vi "GetVariantToDataError.vi"(10 "error close reference":errorcluster, 11 "server":T1={"vi name"="", "VI Refnum"=refnum, "queue"=refnum, "ROS"={"topic port"=0, "Node"="", "topic"="", "type"="", "node port"=0, "error "={"status"=FALSE, "code"=0, "source"=""}, "Direction"=enum."Node", "APIs"=[], "Update (ms)"=1, "write queue"=1}, "notifier"=refnum}) -> ()   [LabVIEW 2012]
uses:
  <userlib>/ROSforLV/ROS/Code/Console/Servers/ServerSubs/ServoInfo.ctl
  <userlib>/ROSforLV/ROS/Code/SubVIs/_ROSControl.ctl
  <userlib>/ROSforLV/ROS/Code/SubVIs/_ROSDirection.ctl
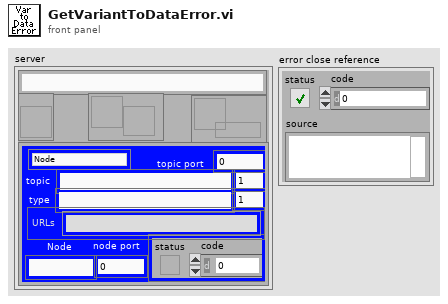
[diagram p1: front panel]
types:
  T1 = typedef "ServoInfo.ctl" = cluster{"vi name":string, "VI Refnum":refnum<vi>, "queue":refnum<queue>, "ROS":T2, "notifier":refnum<notifier>}
  T2 = typedef "_ROSControl.ctl" = cluster{"topic port":u16, "Node":string, "topic":string, "type":string, "node port":u16, "error ":errorcluster, "Direction":T3, "APIs":string[], "Update (ms)":u16, "write queue":u16}
  T3 = typedef "_ROSDirection.ctl" = enum16{"Node", "Publisher", "Subscriber", "Service Client"}
  T4 = enum16{"open", "replace", "create", "open or create", "replace or create", "replace or create with confirmation"}
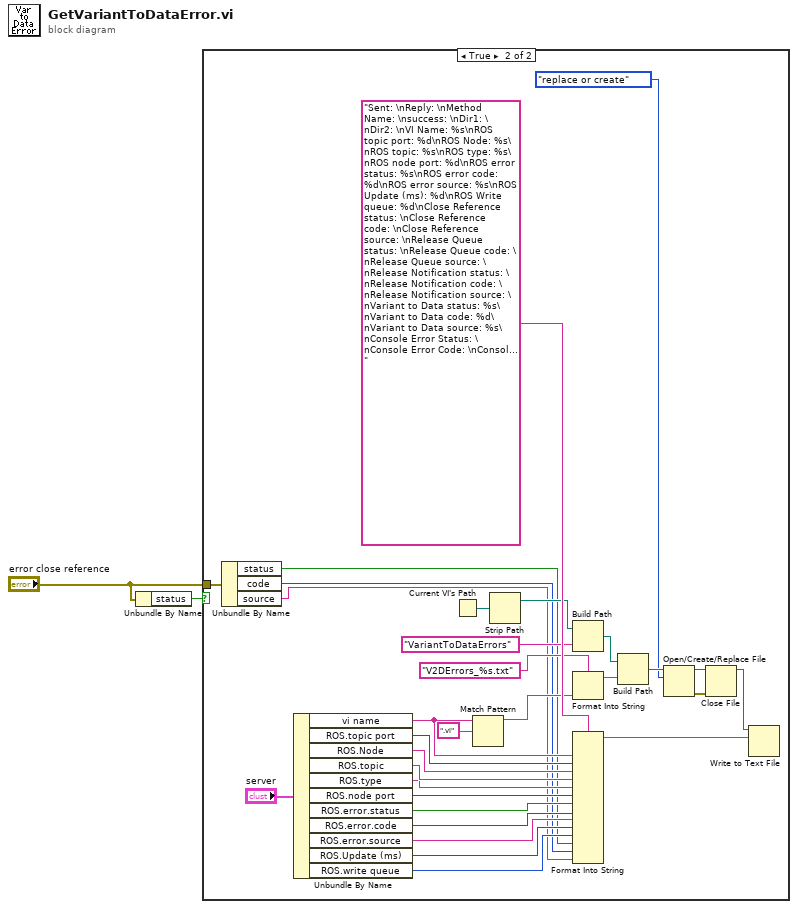
[diagram p0: block diagram]
diagram:
  n1 = Unbundle By Name("error close reference") -> ("status"=w2:bool)
  n2 = case shown="True" w2 {
    tunnel: "error close reference" -> [_ w17]
    frame False {
    }
    frame True {
      n3 = Unbundle By Name(w17) -> ("status"=w5:bool, "code"=w4:i32, "source"=w3:string)
      n4 = Unbundle By Name("server") -> ("vi name"=w16:string, "ROS.topic port"=w15:u16, "ROS.Node"=w14:string, "ROS.topic"=w13:string, "ROS.type"=w12:string, "ROS.node port"=w11:u16, "ROS.error.status"=w10:bool, "ROS.error.code"=w9:i32, "ROS.error.source"=w8:string, "ROS.Update (ms)"=w7:u16, "ROS.write queue"=w6:u16)
      n5 = Current VI's Path() -> (path=w31:path)
      n6 = Match Pattern(string=w16, regular expression=".vi") -> (before substring=w18:string)  [unwired: 1 in, 3 out]
      n7 = Strip Path(path=w31) -> (stripped path=w30:path)  [unwired: 1 out]
      n8 = Build Path(base path=w30, name or relative path="VariantToDataErrors") -> (appended path=w28:path)
      n9 = Format Into String(format string="V2DErrors_%s.txt", w18) -> (resulting string=w21:string)  [unwired: 2 in, 1 out]
      n10 = Format Into String(format string="Sent: \nReply: \nMethod Name: \nsuccess: \nDir1: \nDir2: \nVI Name: %s\nROS topic port: %d\nROS Node: %s\nROS topic: %s\nROS type: %s\nROS node port: %d\nROS error status: %s\nROS error code: %d\nROS error source: %s\nROS Update (ms): %d\nROS Write queue: %d\nClose Reference status: \nClose Reference code: \nClose Reference source: \nRelease Queue status: \nRelease Queue code: \nRelease Queue source: \nRelease Notification status: \nRelease Notification code: \nRelease Notification source: \nVariant to Data status: %s\nVariant to Data code: %d\nVariant to Data source: %s\nConsole Error Status: \nConsole Error Code: \nConsole Error Source: \nTimestamp: \n====", w16, w15, w14, w13, w12, w11, w10, w9, w8, w7, w6, w5, w4, w3) -> (resulting string=w33:string)  [unwired: 2 in, 1 out]
      n11 = Build Path(base path=w28, name or relative path=w21) -> (appended path=w25:path)
      n12 = Open/Create/Replace File(file path (use dialog)=w25, operation (0:open)=T4."replace or create") -> (refnum out=w26:refnum<file>, error out=w27:errorcluster)  [unwired: 4 in, 1 out]
      n13 = Close File(refnum=w26, error in=w27) -> (path=w23:path)  [unwired: 1 out]
      n14 = Write to Text File(file (use dialog)=w23, text=w33) -> ()  [unwired: 2 in, 3 out]
    }
  }
